vi "setTics.vi"(7 "tics":T3={"ticMin"=0.0, "ticStep"=0.0, "ticMax"=0.0, "minorDivsPerMajor"=2, "Mirror tics"=TRUE, "ticSpacing"=enum."Auto Tics"}, 8 "AxisSpan":dbl, 9 "Axis":T2, 11 "String in":string) -> (0 "polarGrid":dbl, 3 "String out":string)   [LabVIEW 2012]
uses:
  tics.ctl
  axisName.ctl
  commandArray.ctl
panel:
  out "Commands":T1
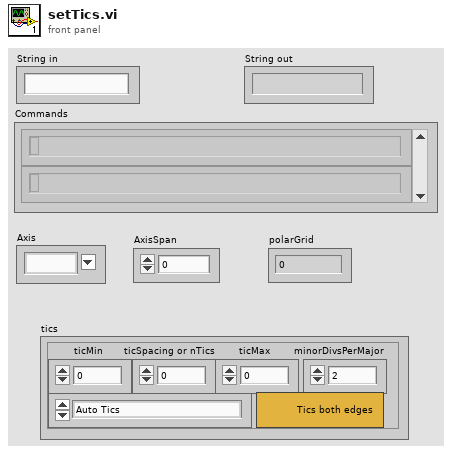
[diagram p1: front panel]
types:
  T1 = typedef "commandArray.ctl" = string[]
  T2 = typedef "axisName.ctl" = string
  T3 = typedef "tics.ctl" = cluster{"ticMin":dbl, "ticStep":dbl, "ticMax":dbl, "minorDivsPerMajor":i32, "Mirror tics":bool, "ticSpacing":enum16{"Auto Tics", "Fixed spacing", "Fixed Minimum and Spacing", "Start, Spacing and Maximum", "Approx n Tics (rounded)"}}
  T4 = enum16{"Auto Tics", "Fixed spacing", "Fixed Minimum and Spacing", "Start, Spacing and Maximum", "Approx n Tics (rounded)"}
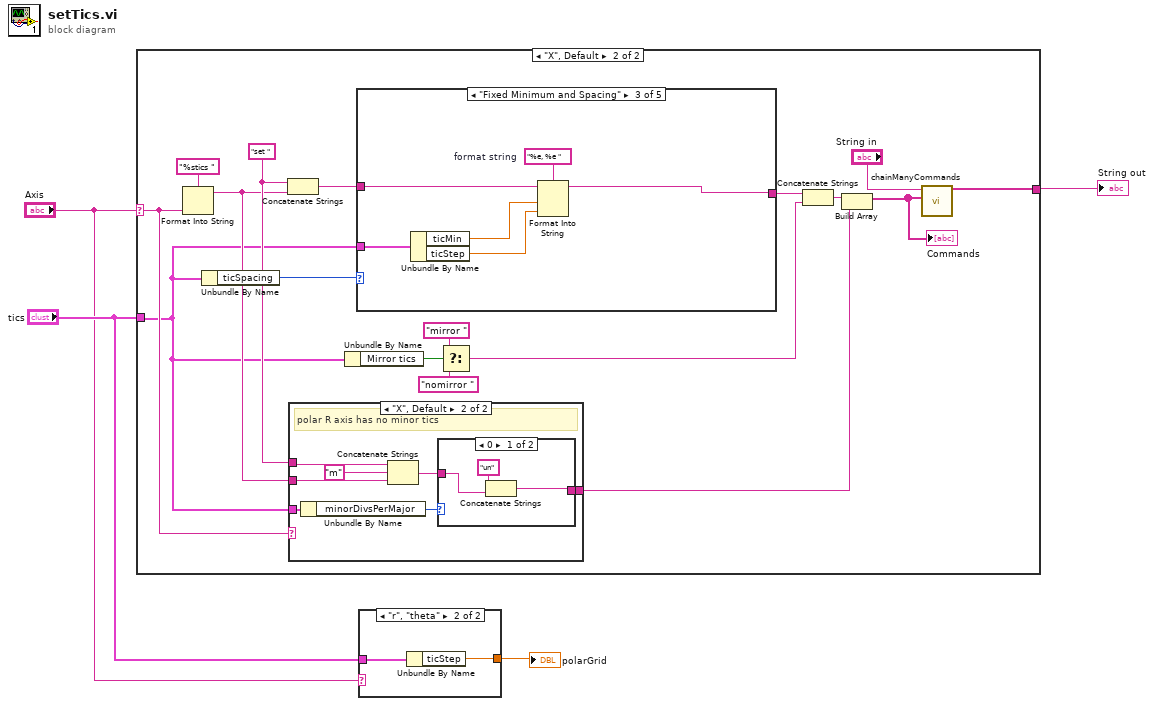
[diagram p0: block diagram]
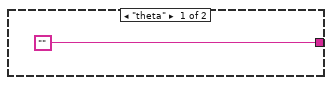
[diagram p2: hidden frame]
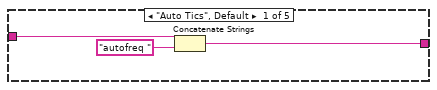
[diagram p3: hidden frame]
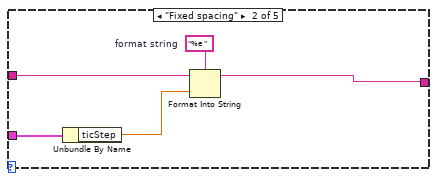
[diagram p4: hidden frame]
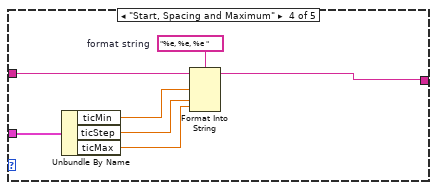
[diagram p5: hidden frame]
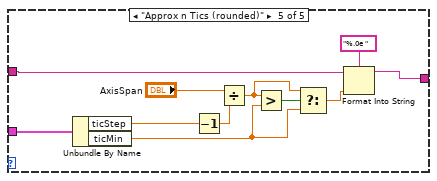
[diagram p6: hidden frame]
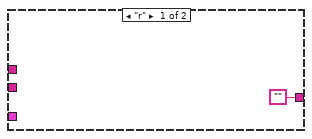
[diagram p7: hidden frame]
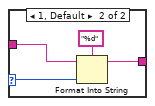
[diagram p8: hidden frame]
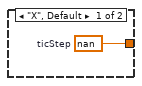
[diagram p9: hidden frame]
diagram:
  n1 = case shown="\"X\", Default" "Axis" {
    selector: "Axis" -> [_ w12]
    tunnel: ["" w17] -> w4
    tunnel: "tics" -> [_ w7]
    frame "theta" {
    }
    frame "X", Default {
      w11 = "set " ("format string")
      n2 = Format Into String(format string="%stics ", w12) -> (resulting string=w10:string)  [unwired: 2 in, 1 out]
      n3 = Unbundle By Name(w7) -> ("ticSpacing"=w6:T4)
      n4 = Concatenate Strings(w11, w10) -> (w9:string)
      n5 = case shown="\"X\", Default" w12 {
        tunnel: w11 -> [_ w61]
        tunnel: w10 -> [_ w60]
        tunnel: ["" w57] -> w14
        tunnel: w7 -> [_ w56]
        frame "r" {
        }
        frame "X", Default {
          # "polar R axis has no minor tics"
          n6 = Unbundle By Name(w56) -> ("minorDivsPerMajor"=w62:i32)
          n7 = Concatenate Strings(w61, "m" ("string"), w60) -> (w58:string)
          n8 = case shown="0" w62 {
            selector: w62 -> [_ w67]
            tunnel: w58 -> [w65 w68]
            tunnel: [w64 w66] -> w57
            frame 0 {
              n9 = Concatenate Strings("un" ("string"), w65) -> (w64:string)
            }
            frame 1, Default {
              n10 = Format Into String(format string="%d", initial string=w68, w67) -> (resulting string=w66:string)  [unwired: 1 in, 1 out]
            }
          }
        }
      }
      n11 = Unbundle By Name(w7) -> ("Mirror tics"=w19:bool)
      n12 = case shown="\"Fixed Minimum and Spacing\"" w6 {
        tunnel: w9 -> [w25 w30 w36 w43 w44]
        tunnel: [w24 w26 w32 w39 w54] -> w8
        tunnel: w7 -> [_ w29 w35 w42 w53]
        frame "Auto Tics", Default {
          n13 = Concatenate Strings(w25, "autofreq " ("string")) -> (w24:string)
        }
        frame "Fixed spacing" {
          w27 = "%e "  # format string
          n14 = Unbundle By Name(w29) -> ("ticStep"=w28:dbl)
          n15 = Format Into String(format string=w27, initial string=w30, w28) -> (resulting string=w26:string)  [unwired: 1 in, 1 out]
        }
        frame "Fixed Minimum and Spacing" {
          w33 = "%e, %e "  # format string
          n16 = Unbundle By Name(w35) -> ("ticMin"=w34:dbl, "ticStep"=w31:dbl)
          n17 = Format Into String(format string=w33, initial string=w36, w34, w31) -> (resulting string=w32:string)  [unwired: 1 in, 1 out]
        }
        frame "Start, Spacing and Maximum" {
          w40 = "%e, %e, %e "  # format string
          n18 = Unbundle By Name(w42) -> ("ticMin"=w41:dbl, "ticStep"=w38:dbl, "ticMax"=w37:dbl)
          n19 = Format Into String(format string=w40, initial string=w43, w41, w38, w37) -> (resulting string=w39:string)  [unwired: 1 in, 1 out]
        }
        frame "Approx n Tics (rounded)" {
          n20 = Unbundle By Name(w53) -> ("ticStep"=w46:dbl, "ticMin"=w47:dbl)
          n21 = Decrement(x=w46) -> (x-1=w48:dbl)
          n22 = Divide(x="AxisSpan", y=w48) -> (x/y=w51:dbl)
          n23 = Greater?(x=w51, y=w47) -> (0:w50:bool)
          n24 = Select(t=w51, s=w50, f=w47) -> (s? t:f=w52:dbl)
          n25 = Format Into String(format string="%.0e ", initial string=w44, w52) -> (resulting string=w54:string)  [unwired: 1 in, 1 out]
        }
      }
      n26 = Select(t="mirror ", s=w19, f="nomirror ") -> (s? t:f=w22:string)
      n27 = Concatenate Strings(w8, w22) -> (w15:string)
      n28 = Build Array(w15, w14) -> (w13:string[])
      "Commands" <- w13
      n29 = call "chainManyCommands.vi"("CommandArray"=w13, "String in in"="String in") -> ("String out"=w17:string)  [unwired: 9 in]
    }
  }
  "String out" <- w4
  n30 = case shown="\"r\", \"theta\"" "Axis" {
    tunnel: "tics" -> [_ w72]
    tunnel: [w70 w71] -> w2
    frame "X", Default {
      w70 = nan  # ticStep
    }
    frame "r", "theta" {
      n31 = Unbundle By Name(w72) -> ("ticStep"=w71:dbl)
    }
  }
  "polarGrid" <- w2
